vi "initialise.vi"(8 "error in (no error)":errorcluster, 11 "Pixelfly in":refnum<class "Pixelfly.lvclass">) -> (0 "error out":errorcluster, 3 "Pixelfly out":refnum<class "Pixelfly.lvclass">)   [LabVIEW 2009, in "Hardware.lvlib" / "Channels.lvlib" / "Pixelfly.lvclass"]
uses:
  Pixelfly.lvclass
  Pixelfly.lvclass/Pixelfly.ctl
  Camera.lvclass
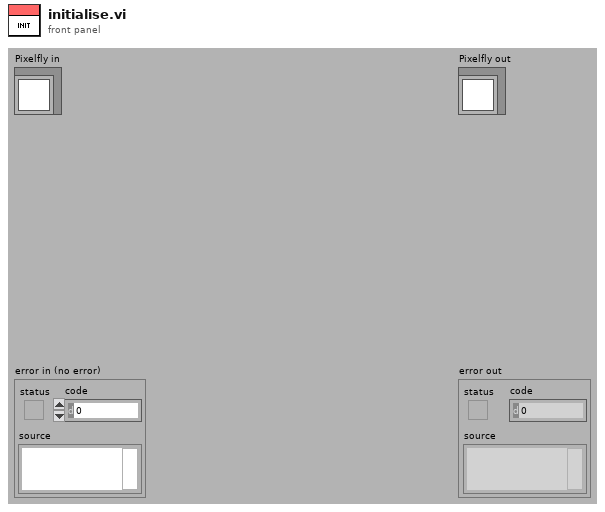
[diagram p1: front panel]
types:
  T1 = cluster{"Message":enum16{"Idle", "initialise", "configureAcquisition", "setTemperature", "getTemperature", "start", "stop", "sendImage", "close", "error", "ExitApp", "getAcquisitionStatus"}, "Data":variant}
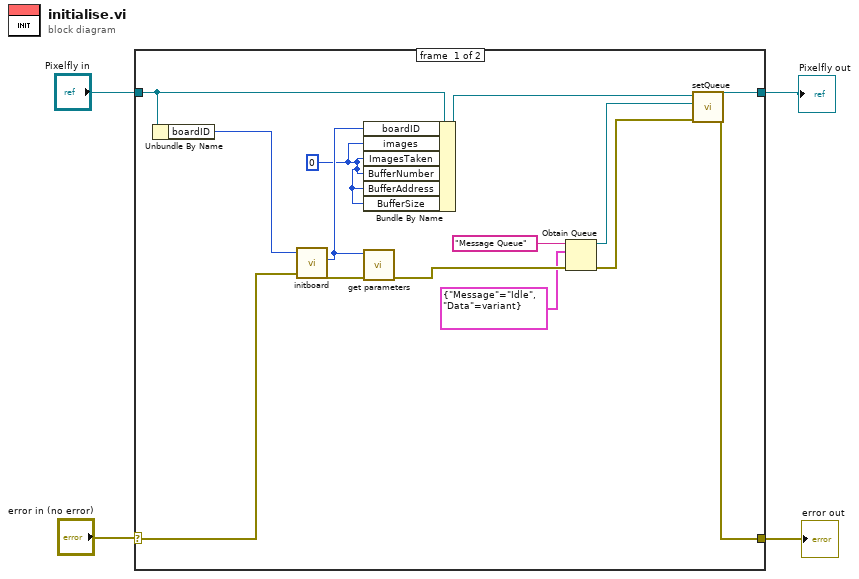
[diagram p0: block diagram]
diagram:
  n1 = case shown="No Error" "error in (no error)" {
    selector: "error in (no error)" -> [w15 w19]
    tunnel: "Pixelfly in" -> [w12 w20]
    tunnel: [w11 w20] -> w2
    tunnel: [w8 w19] -> w1
    frame #0 {
      w6 = 0
      n2 = Unbundle By Name(w12) -> ("boardID"=w17:i32)
      n3 = call <instrlib>:"initboard.vi"("boardid in"=w17, "error in (no error)"=w15) -> ("boardid"=w16:i32, "error out"=w18:errorcluster)  [unwired: 2 in, 1 out]
      n4 = Bundle By Name(cluster=w12, "boardID"=w16, "images"=w6, "ImagesTaken"=w6, "BufferNumber"=w6, "BufferAddress"=w6, "BufferSize"=w6) -> (w10:refnum<class "Pixelfly.lvclass">)
      n5 = call <instrlib>:"get parameters.vi"("error in (no error)"=w18, "Handle in"=w16) -> ("error out"=w14:errorcluster)  [unwired: 2 in, 3 out]
      n6 = Obtain Queue(name (unnamed)="Message Queue" ("Queue Name"), element data type=T1 {"Message"=enum."Idle", "Data"=variant}, error in (no error)=w14) -> (queue out=w7:refnum<queue>, error out=w9:errorcluster)  [unwired: 2 in, 1 out]
      n7 = call "setQueue.vi"("error in (no error)"=w9, "queue"=w7, "Camera in"=w10) -> ("error out"=w8:errorcluster, "Camera out"=w11:refnum<class "Pixelfly.lvclass">)  [unwired: 7 in]
    }
    frame #1 {
    }
  }
  "error out" <- w1
  "Pixelfly out" <- w2
